vi "zurich_lock_in_Open_Queue_1.vi"(8 "error in (no error)":errorcluster) -> (0 "error out":errorcluster, 3 "queue out":refnum<queue>)   [LabVIEW 2019]
uses:
  zurich_lock_in/zurichinstMonitor.ctl
  Global/Global Variables/Queues_global.vi
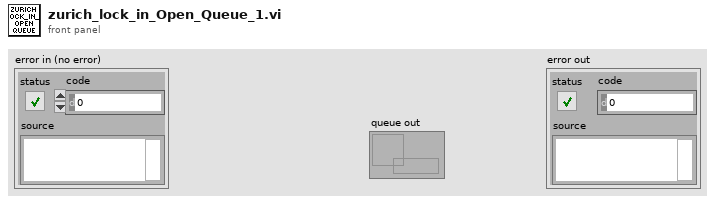
[diagram p1: front panel]
types:
  T1 = typedef "zurichinstMonitor.ctl" = cluster{"Dmod 1 X":dbl, "Dmod 1 Y":dbl, "Dmod 1 R":dbl, "Dmod 1 Theta":dbl, "Update Oscillators":bool, "Dmod 2 X":dbl, "Dmod 2 R":dbl, "Dmod 2 Y":dbl, "Dmod 2 Theta":dbl}
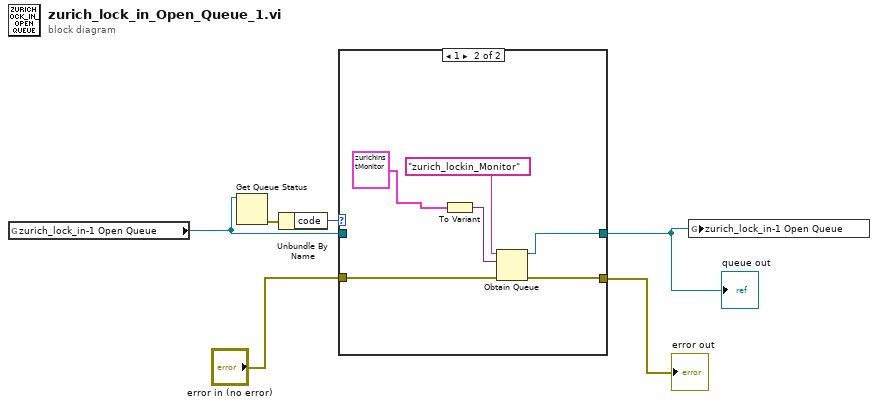
[diagram p0: block diagram]
diagram:
  n1 = global read "Queues_global.vi" "zurich_lock_in-1 Open Queue"() -> (w4:refnum<queue>)
  n2 = Get Queue Status(queue=w4) -> (error out=w6:errorcluster)  [unwired: 2 in, 7 out]
  n3 = Unbundle By Name(w6) -> ("code"=w5:i32)
  n4 = case shown="1" w5 {
    tunnel: [w8 w12] -> w3
    tunnel: w4 -> [w8 _]
    tunnel: "error in (no error)" -> [w7 w11]
    tunnel: [w7 w10] -> w1
    frame 0, Default {
    }
    frame 1 {
      n5 = To Variant(anything=T1 {"Dmod 1 X"=0.0, "Dmod 1 Y"=0.0, "Dmod 1 R"=0.0, "Dmod 1 Theta"=0.0, "Update Oscillators"=FALSE, "Dmod 2 X"=0.0, "Dmod 2 R"=0.0, "Dmod 2 Y"=0.0, "Dmod 2 Theta"=0.0} ("Zurich-Lock-In Monitor")) -> (Variant=w13:variant)
      n6 = Obtain Queue(name (unnamed)="zurich_lockin_Monitor", element data type=w13, error in (no error)=w11) -> (queue out=w12:refnum<queue>, error out=w10:errorcluster)  [unwired: 2 in, 1 out]
    }
  }
  "queue out" <- w3
  "error out" <- w1
  n7 = global write "Queues_global.vi" "zurich_lock_in-1 Open Queue"(w3) -> ()
